vi "Lookup Group State Indices.vi"(7 "Map":map{string, i32}(c390), 8 "error in (no error)":errorcluster, 11 "Log Manager Module in":refnum<class "Log Manager Module.lvclass">) -> (0 "error out":errorcluster, 2 "Group State Indices":i32[](array[numeric]), 3 "Log Manager Module out":refnum<class "Log Manager Module.lvclass">)   [LabVIEW 2020, in "VolatusData.lvlib" / "Log Manager Module.lvclass"]
uses:
  Log Manager Module.lvclass
  Log Manager Module.lvclass/Log Manager Module.ctl
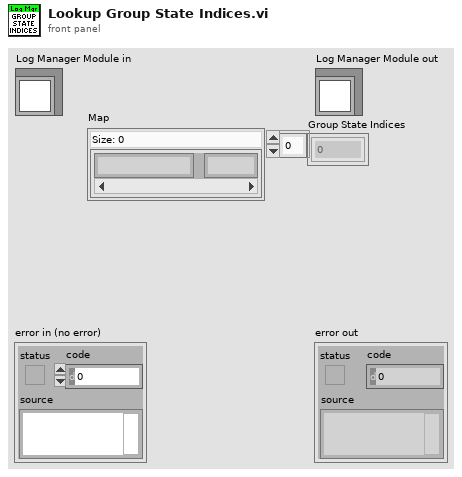
[diagram p1: front panel]
types:
  T1 = typedef "VolatusData.lvlib/Log Manager Module.lvclass/Group Info.ctl" = cluster{"Name":string, "Loggers":map{string, T2}}
  T2 = typedef "VolatusData.lvlib/Log Manager Module.lvclass/Logger.ctl" = cluster{"ID":string, "MsgQ":refnum<class "MessageQ.lvclass">, "State":T3, "Group":string}
  T3 = typedef "VolatusData.lvlib/Logger State.ctl" = enum16{"Unknown", "Idle", "Preparing", "Ready", "Logging", "Stopping"}
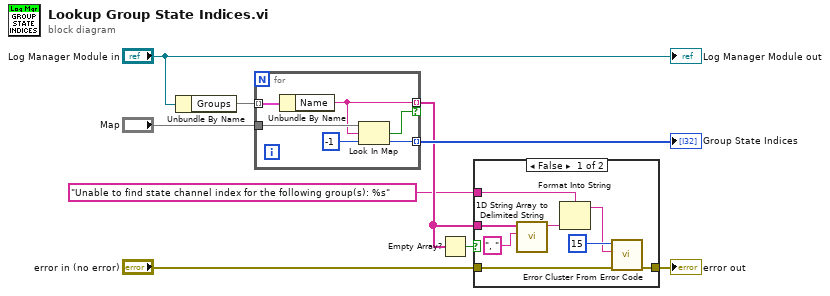
[diagram p0: block diagram]
diagram:
  n1 = Unbundle By Name("Log Manager Module in") -> ("Groups"=w7:map{string, T1})
  n2 = for {
    tunnel: "Map" -> [w14]
    tunnel: w7 -> [w15] mode=indexing
    tunnel: [w12] -> w6 mode=indexing
    tunnel: [w11] -> w2 mode=indexing if=w10
    n3 = Unbundle By Name(w15) -> ("Name"=w11:string)
    n4 = Look In Map(map=w14, key=w11, default value=-1) -> (key not found?=w10:bool, value=w12:i32)
  }
  "Group State Indices" <- w6
  n5 = Empty Array?(array=w2) -> (empty?=w5:bool)
  n6 = case shown="False" w5 {
    tunnel: [w22 w24] -> w4
    tunnel: "error in (no error)" -> [w23 w24]
    tunnel: w2 -> [w20 _]
    tunnel: "Unable to find state channel index for the following group(s): %s" -> [w16 _]
    frame False {
      n7 = call <vilib>:"1D String Array to Delimited String.vi"("delimiter"=", ", "string array"=w20) -> ("delimited string"=w18:string)  [unwired: 9 in]
      n8 = Format Into String(format string=w16, w18) -> (resulting string=w17:string)  [unwired: 2 in, 1 out]
      n9 = call <vilib>:"Error Cluster From Error Code.vi"("error in (no error)"=w23, "error message (\"\")"=w17, "error code (0)"=15) -> ("error out"=w22:errorcluster)  [unwired: 6 in]
    }
    frame True {
    }
  }
  "error out" <- w4
  "Log Manager Module out" <- "Log Manager Module in"
